vi "GetRandomString.vi"(8 "error in (no error)":errorcluster, 11 "Generator in":refnum<class "Generator.lvclass">) -> (0 "error out":errorcluster, 3 "Generator out":refnum<class "Generator.lvclass">)   [LabVIEW 2014, in "Generator.lvlib" / "Generator.lvclass"]
uses:
  Generator.lvclass
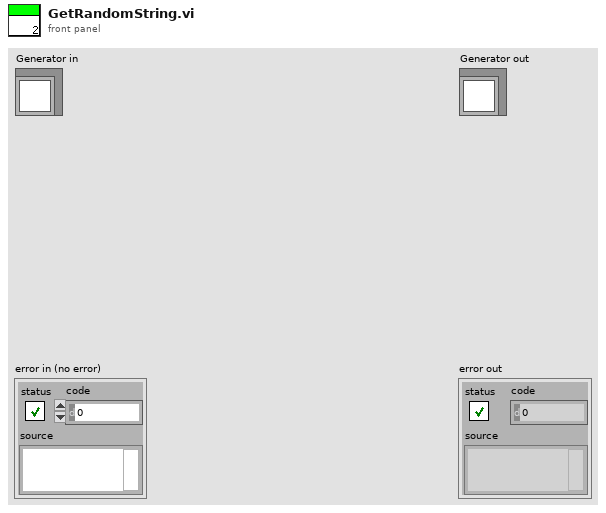
[diagram p1: front panel]
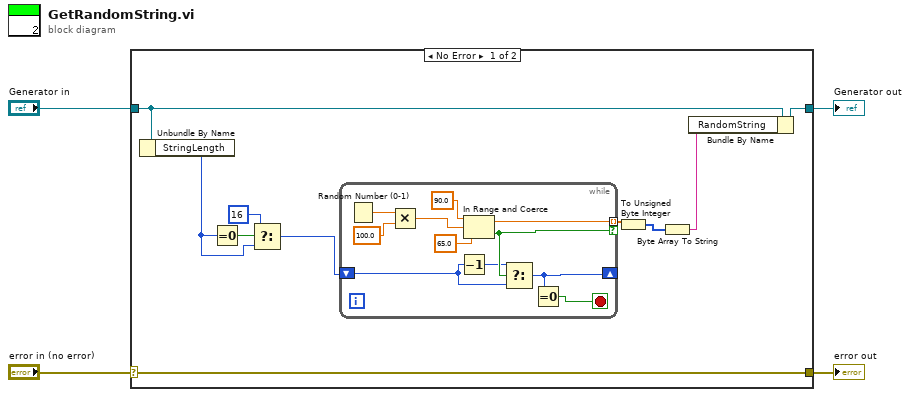
[diagram p0: block diagram]
diagram:
  n1 = case shown="No Error" "error in (no error)" {
    selector: "error in (no error)" -> [w14 w27]
    tunnel: [w14 w27] -> w3
    tunnel: [w11 w26] -> w1
    tunnel: "Generator in" -> [w9 w26]
    frame No Error {
      n2 = Unbundle By Name(w9) -> ("StringLength"=w7:i32)
      n3 = Equal To 0?(x=w7) -> (x = 0?=w8:bool)
      n4 = Select(t=16, s=w8, f=w7) -> (s? t:f=w5:i32)
      n5 = while {
        tunnel: [w20] -> w13 mode=indexing if=w19
        shift-right: [w16] -> _
        shift-left: w5 -> [w17]
        stop <- w15 stop-if-true
        n6 = Random Number (0-1)() -> (number: 0 to 1=w25:dbl)
        n7 = Multiply(x=w25, y=100.0) -> (x*y=w24:dbl)
        n8 = Decrement(x=w17) -> (x-1=w18:i32)
        n9 = In Range and Coerce(upper limit=90.0, x=w24, lower limit=65.0) -> (coerced(x)=w20:dbl, In Range?=w19:bool)
        n10 = Select(t=w18, s=w19, f=w17) -> (s? t:f=w16:i32)
        n11 = Equal To 0?(x=w16) -> (x = 0?=w15:bool)
      }
      n12 = To Unsigned Byte Integer(number=w13) -> (unsigned 8bit integer=w12:u8[])
      n13 = Byte Array To String(unsigned byte array=w12) -> (string=w10:string)
      n14 = Bundle By Name(cluster=w9, "RandomString"=w10) -> (w11:refnum<class "Generator.lvclass">)
    }
    frame Error {
    }
  }
  "error out" <- w3
  "Generator out" <- w1
